vi "Make Sound.vi"(8 "error in (no error)":errorcluster, 11 "Chicken in":refnum<class "Chicken.lvclass">) -> (0 "error out":errorcluster, 3 "Chicken out":refnum<class "Chicken.lvclass">)   [LabVIEW 2024, in "Chicken.lvclass"]
doc: "本VI是为《我和LabVIEW》一书编写的示例。\n关于本书的介绍请参考网页：\nhttp://ruanqizhen.spaces.live.com/blog/cns!5852D4F797C53FB6!4310.entry"
uses:
  Chicken.lvclass
  Animal/Animal.lvclass
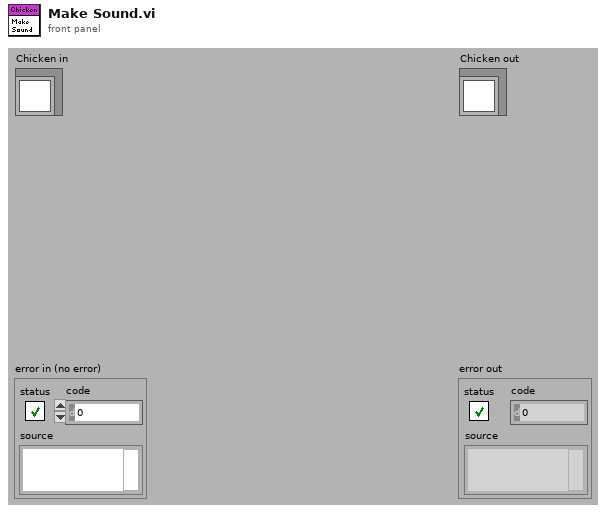
[diagram p1: front panel]
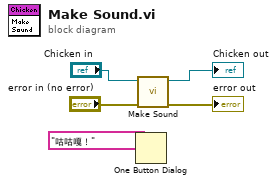
[diagram p0: block diagram]
diagram:
  n1 = One Button Dialog(message="咕咕嘎！") -> ()  [unwired: 2 out]
  n2 = call-parent "Make Sound.vi"("error in (no error)"="error in (no error)", "Animal in"="Chicken in") -> ("error out"=→"error out":errorcluster, "Animal out"=→"Chicken out":refnum<class "Chicken.lvclass">)  [unwired: 8 out]
